vi "Smooth.vi"(9 "Clip end ramps":bool, 10 "Smooth point width":dbl=32.0, 11 "Input":dbl[](array[numeric])) -> (2 "Clip length":i32, 3 "Output":dbl[](array[numeric]))   [LabVIEW 2021]
uses:
  <vilib>/Analysis/3filter.llb/Filter Passband Type.ctl
  <vilib>/Analysis/3filter.llb/Butterworth Filter (DBL).vi
  <vilib>/Analysis/NI_AALBase.lvlib
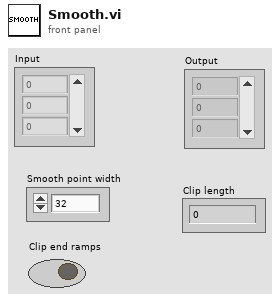
[diagram p1: front panel]
types:
  T1 = typedef "NI_AALBase.lvlib/Filter Passband Type.ctl" = enum32{"Lowpass", "Highpass", "Bandpass", "Bandstop"}
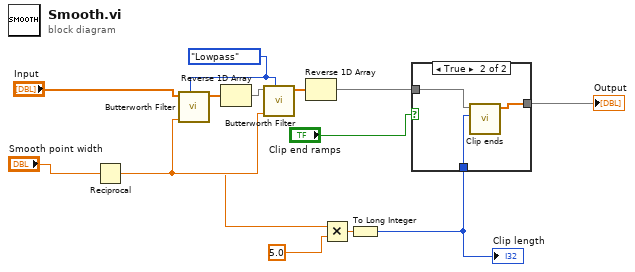
[diagram p0: block diagram]
diagram:
  w9 = Filter_Passband_Type."Lowpass" ("filter type")
  n1 = Reciprocal(x="Smooth point width") -> (1/x=w8:dbl)
  n2 = call-poly <vilib>:"Butterworth Filter.vi"("filter type"=w9, "low cutoff freq: fl"=w8, "X"="Input") -> ("Filtered X"=w13:dbl[])  [unwired: 5 in, 1 out]
  n3 = Reverse 1D Array(array=w13) -> (reversed array=w12:dbl[])
  n4 = call-poly <vilib>:"Butterworth Filter.vi"("filter type"=w9, "low cutoff freq: fl"=w8, "X"=w12) -> ("Filtered X"=w11:dbl[])  [unwired: 5 in, 1 out]
  n5 = Reverse 1D Array(array=w11) -> (reversed array=w5:dbl[])
  n6 = Multiply(x="Smooth point width", y=5.0) -> (x*y=w2:dbl)
  n7 = To Long Integer(number=w2) -> (32bit integer=w1:i32)
  "Clip length" <- w1
  n8 = case shown="True" "Clip end ramps" {
    tunnel: w5 -> [w14 w17]
    tunnel: [w14 w16] -> w4
    tunnel: w1 -> [_ w15]
    frame False {
    }
    frame True {
      n9 = call "Clip ends.vi"("Clip length"=w15, "Input"=w17) -> ("Output"=w16:dbl[])  [unwired: 9 in]
    }
  }
  "Output" <- w4
